vi "FPGA.vi"() -> ()   [LabVIEW 2019]
uses:
  <vilib>/rvi/Emulation/niFpgaGetClockAttributes.vi
  <vilib>/rvi/Emulation/niFpgaSctlEmulationGetInTimedLoop.vi
  <vilib>/rvi/Emulation/niFpgaEmulationReportErrorSimple.vi
  <vilib>/rvi/eio/common/nirviEmuTemplateMethod_errors.vi
  <vilib>/rvi/Memory/Memory_Emulation/nirvimemoryFastEmulation.vi
  <vilib>/rvi/Memory/Memory_Emulation/nirvimemoryEmulation.vi
  <vilib>/rvi/Emulation/niFpgaEmulationIsFPGAContextNoSignature.vi
  <vilib>/rvi/DataTransferAndStorage/Container/Common/niFpgaContainerGetUniqueNameForEmu.vi
  <vilib>/rvi/Emulation/niFpgaProcessEmulError.vi
  <vilib>/rvi/errors/nirviReportUnexpectedCaseInternalError (U32).vi
  <vilib>/rvi/DataTransferAndStorage/Container/Common/niFpgaContainerExecOnDevCompGetState.vi
  <vilib>/rvi/Memory/Memory_Emulation/niFpgaMemoryEmulationCacheClearOnFirstRun.vi
  <vilib>/rvi/Memory/Memory_Emulation/nirvimemoryEmulationManagerCache_MakeExclusive.vi
  <vilib>/rvi/Memory/Memory_Emulation/niFpgaMemoryEmulationValidateCache.vi
  <vilib>/rvi/Memory/Memory_Emulation/nirvimemoryEmulationManagerCache_InsertValue.vi
  <vilib>/Utility/error.llb/Clear Errors.vi
  <vilib>/rvi/Memory/Memory_Emulation/nirvimemoryEmulationManagerCache_ReleaseExclusive.vi
  <vilib>/rvi/Memory/Memory_Emulation/nirvimemoryEmulationManagerCache_GetValue.vi
  <vilib>/rvi/Memory/Memory_Emulation/nirvimemoryEmulationManagerCache_SetValue.vi
  <vilib>/rvi/Emulation/niFpgaSctlEmulationResourceMgr.vi
  <vilib>/rvi/Emulation/niFpgaCriticalErrorInLSC.vi
  <vilib>/eio/EIONode/EIONode.xnode
  <vilib>/rvi/DataTransferAndStorage/Container/XNode/niFpgaContainer.xnode
  <vilib>/rvi/Memory/Memory_Emulation/niFpgaMemoryEmulationRefIn.vi
panel:
  out "MeanZ":fxp<+/-,32,32>
  out "MeanY":fxp<+/-,32,32>
  out "MeanX":fxp<+/-,32,32>
  in  "Z Threshold":i16
  in  "Y Threshold":i16
  in  "X Threshold":i16
  out "Z MAX":i16
  out "Y MAX":i16
  out "X MAX":i16
  out "Z Acceleration":i16
  out "Y Acceleration":i16
  out "X Acceleration":i16
  in  "Dzielnik":i64
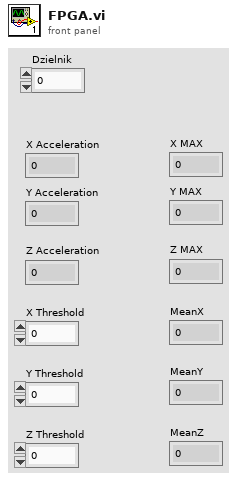
[diagram p1: front panel]
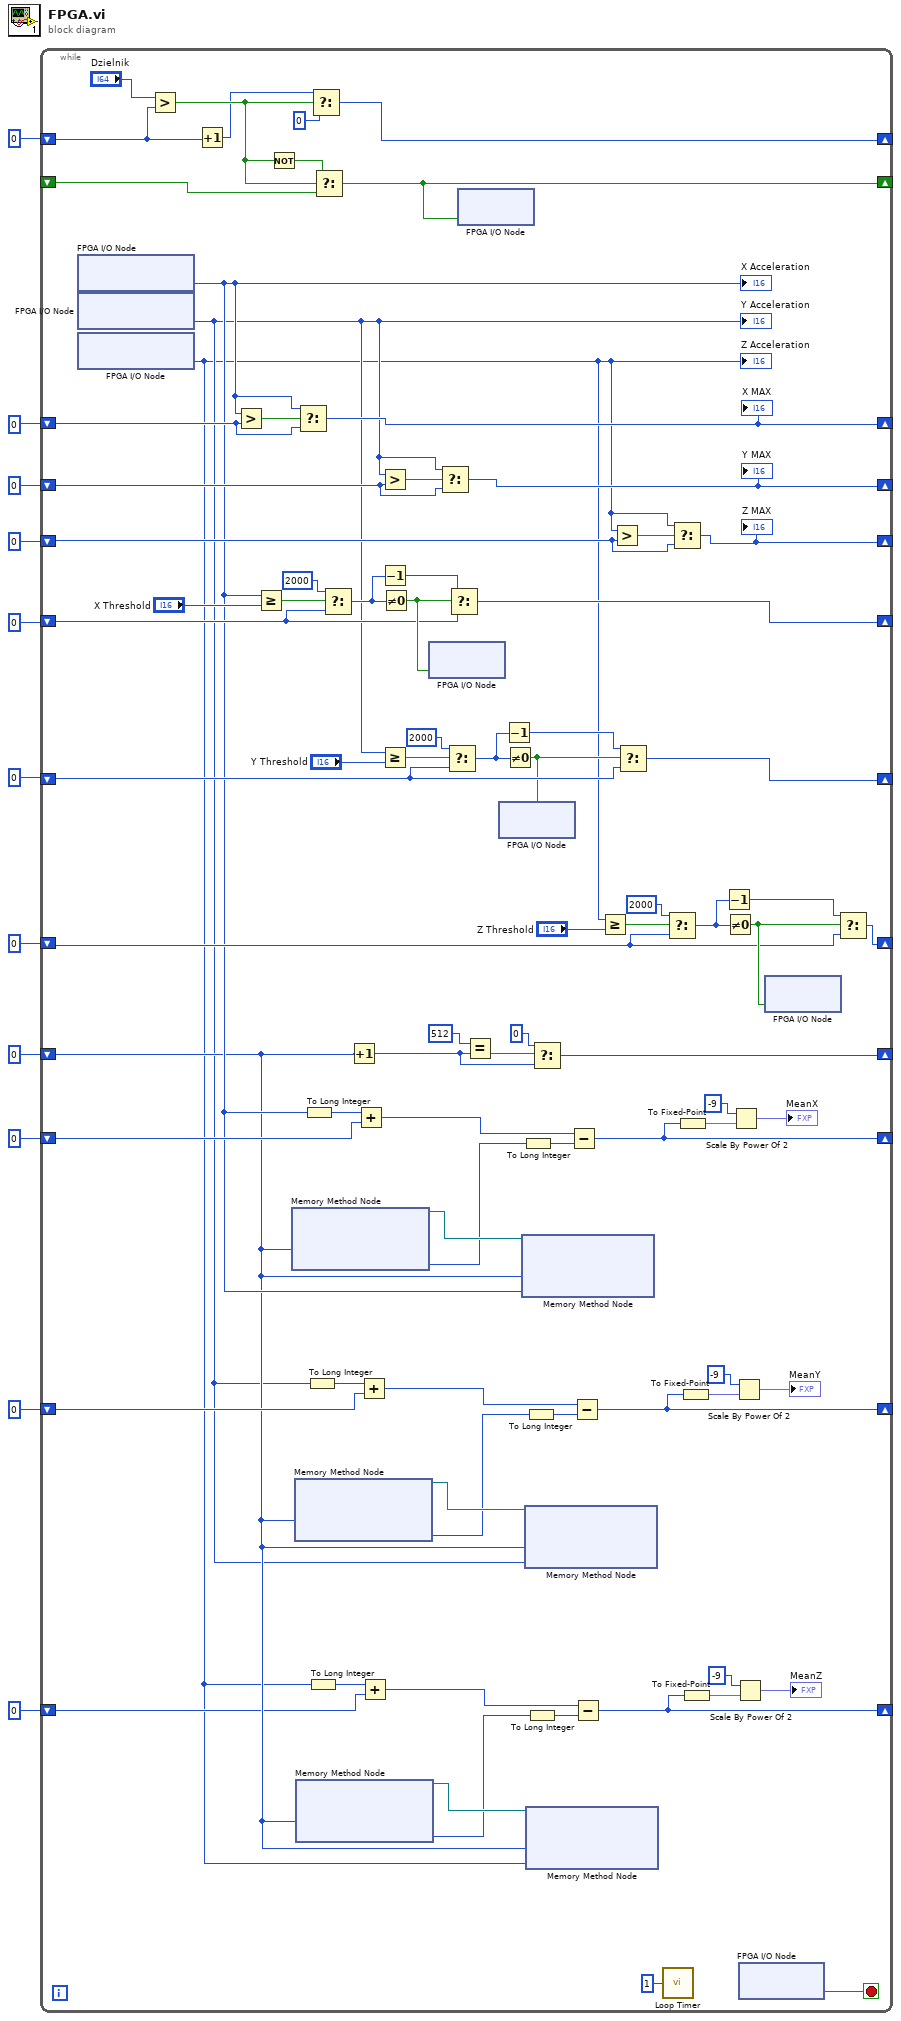
[diagram p0: block diagram]
diagram:
  n1 = while {
    shift-right: [w88] -> _
    shift-left: _ -> [w91]
    shift-right: [w92] -> _
    shift-left: i64 0 -> [w93]
    shift-right: [w81] -> _
    shift-left: i16 0 -> [w86]
    shift-right: [w80] -> _
    shift-left: i16 0 -> [w84]
    shift-right: [w79] -> _
    shift-left: i16 0 -> [w82]
    shift-right: [w70] -> _
    shift-left: i16 0 -> [w64]
    shift-right: [w62] -> _
    shift-left: i16 0 -> [w63]
    shift-right: [w54] -> _
    shift-left: i16 0 -> [w55]
    shift-right: [w43] -> _
    shift-left: u32 0 ("t") -> [w17]
    shift-right: [w39] -> _
    shift-left: 0 -> [w52]
    shift-right: [w26] -> _
    shift-left: 0 -> [w27]
    shift-right: [w14] -> _
    shift-left: 0 -> [w15]
    stop <- w53 stop-if-true
    n2 = xnode "FPGA I/O Node"() -> ("AccelerationX"=w48:i16)  [unwired: 1 in, 1 out]
    "X Acceleration" <- w48
    n3 = xnode "FPGA I/O Node"() -> ("AccelerationY"=w13:i16)  [unwired: 1 in, 1 out]
    "Y Acceleration" <- w13
    n4 = xnode "FPGA I/O Node"() -> ("AccelerationZ"=w12:i16)  [unwired: 1 in, 1 out]
    "Z Acceleration" <- w12
    n5 = Greater?(x="Dzielnik", y=w93) -> (0:w89:bool)
    n6 = Increment(x=w93) -> (x+1=w77:i64)
    n7 = Greater?(x=w48, y=w86) -> (0:w87:bool)
    n8 = Greater Or Equal?(x=w48, y="X Threshold") -> (x >= y?=w75:bool)
    n9 = Not(x=w89) -> (.not. x?=w90:bool)
    n10 = xnode ("Memory Method Node")("Address"=w17) -> ("Data"=w49:i16, "Memory Out"=w51:refnum<k21>)  [unwired: 1 in]
    n11 = xnode ("Memory Method Node")("Address"=w17) -> ("Data"=w34:i16, "Memory Out"=w36:refnum<k21>)  [unwired: 1 in]
    n12 = xnode ("Memory Method Node")("Address"=w17) -> ("Data"=w23:i16, "Memory Out"=w25:refnum<k21>)  [unwired: 1 in]
    n13 = Select(t=w48, s=w87, f=w86) -> (s? t:f=w81:i16)
    "X MAX" <- w81
    n14 = To Long Integer(number=w48) -> (32bit integer=w38:i32)
    n15 = To Long Integer(number=w13) -> (32bit integer=w30:i32)
    n16 = To Long Integer(number=w12) -> (32bit integer=w19:i32)
    n17 = Select(t=w77, s=w89, f=i64 0) -> (s? t:f=w92:i64)
    n18 = Select(t=w90, s=w89, f=w91) -> (s? t:f=w88:bool)
    n19 = Select(t=i16 2000, s=w75, f=w64) -> (s? t:f=w72:i16)
    n20 = Increment(x=w17) -> (x+1=w41:u32)
    n21 = Add(x=w38, y=w52) -> (x+y=w50:i32)
    n22 = Add(x=w30, y=w27) -> (x+y=w35:i32)
    n23 = Add(x=w19, y=w15) -> (x+y=w24:i32)
    n24 = Greater?(x=w13, y=w84) -> (0:w85:bool)
    n25 = Decrement(x=w72) -> (x-1=w71:i16)
    n26 = Greater Or Equal?(x=w13, y="Y Threshold") -> (x >= y?=w68:bool)
    n27 = Not Equal To 0?(x=w72) -> (x != 0?=w69:bool)
    n28 = xnode "FPGA I/O Node"("LED1"=w69) -> ()  [unwired: 1 in, 1 out]
    n29 = Select(t=w13, s=w85, f=w84) -> (s? t:f=w80:i16)
    "Y MAX" <- w80
    n30 = Select(t=i16 2000, s=w68, f=w63) -> (s? t:f=w66:i16)
    n31 = Select(t=w71, s=w69, f=w64) -> (s? t:f=w70:i16)
    n32 = xnode "FPGA I/O Node"("LED0"=w88) -> ()  [unwired: 1 in, 1 out]
    n33 = Equal?(x=u32 512 ("t"), y=w41) -> (x = y?=w44:bool)
    n34 = Decrement(x=w66) -> (x-1=w65:i16)
    n35 = Not Equal To 0?(x=w66) -> (x != 0?=w61:bool)
    n36 = xnode "FPGA I/O Node"("LED2"=w61) -> ()  [unwired: 1 in, 1 out]
    n37 = xnode ("Memory Method Node")("Address"=w17, "Data"=w48, "Memory In"=w51) -> ()  [unwired: 1 out]
    n38 = To Long Integer(number=w49) -> (32bit integer=w37:i32)
    n39 = xnode ("Memory Method Node")("Address"=w17, "Data"=w13, "Memory In"=w36) -> ()  [unwired: 1 out]
    n40 = To Long Integer(number=w34) -> (32bit integer=w29:i32)
    n41 = xnode ("Memory Method Node")("Address"=w17, "Data"=w12, "Memory In"=w25) -> ()  [unwired: 1 out]
    n42 = To Long Integer(number=w23) -> (32bit integer=w18:i32)
    n43 = Select(t=u32 0, s=w44, f=w41) -> (s? t:f=w43:u32)
    n44 = Subtract(x=w50, y=w37) -> (x-y=w39:i32)
    n45 = Subtract(x=w35, y=w29) -> (x-y=w26:i32)
    n46 = Subtract(x=w24, y=w18) -> (x-y=w14:i32)
    n47 = Greater Or Equal?(x=w12, y="Z Threshold") -> (x >= y?=w60:bool)
    n48 = Greater?(x=w12, y=w82) -> (0:w83:bool)
    n49 = Select(t=w65, s=w61, f=w63) -> (s? t:f=w62:i16)
    n50 = call "Loop Timer"("Count(mSec)"=u8 1) -> ()  [unwired: 1 out]
    n51 = Select(t=i16 2000, s=w60, f=w55) -> (s? t:f=w58:i16)
    n52 = Select(t=w12, s=w83, f=w82) -> (s? t:f=w79:i16)
    "Z MAX" <- w79
    n53 = To Fixed-Point(number=w39) -> (fixed-point=w40:fxp<+/-,32,32>)  [unwired: 1 in]
    n54 = To Fixed-Point(number=w26) -> (fixed-point=w31:fxp<+/-,32,32>)  [unwired: 1 in]
    n55 = To Fixed-Point(number=w14) -> (fixed-point=w20:fxp<+/-,32,32>)  [unwired: 1 in]
    n56 = Decrement(x=w58) -> (x-1=w57:i16)
    n57 = Not Equal To 0?(x=w58) -> (x != 0?=w56:bool)
    n58 = Scale By Power Of 2(n=-9, x=w40) -> (x*2^n=→"MeanX":fxp<+/-,32,32>)
    n59 = Scale By Power Of 2(n=-9, x=w31) -> (x*2^n=→"MeanY":fxp<+/-,32,32>)
    n60 = Scale By Power Of 2(n=-9, x=w20) -> (x*2^n=→"MeanZ":fxp<+/-,32,32>)
    n61 = xnode "FPGA I/O Node"() -> ("Button0"=w53:bool)  [unwired: 1 in, 1 out]
    n62 = xnode "FPGA I/O Node"("LED3"=w56) -> ()  [unwired: 1 in, 1 out]
    n63 = Select(t=w57, s=w56, f=w55) -> (s? t:f=w54:i16)
  }
